vi "RunOperation.vi"(10 "Inputs":string[](array[string]), 11 "RunVIAnalyzer in":refnum<class "RunVIAnalyzer.lvclass">) -> (1 "Output/Failure":string, 2 "CLI Process Return Code":i32, 3 "RunVIAnalyzer out":refnum<class "RunVIAnalyzer.lvclass">)   [LabVIEW 2014, in "RunVIAnalyzer.lvclass"]
uses:
  RunVIAnalyzer.lvclass
  RunVIAnalyzer.lvclass/RunVIAnalyzer.ctl
  <vilib>/addons/analyzer/NI_VIAnalyzerTKVIs.lvlib
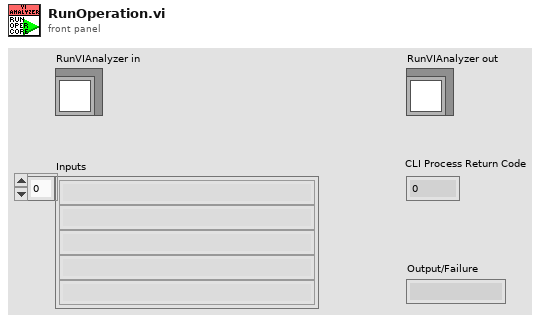
[diagram p1: front panel]
types:
  T1 = typedef "VIAnCtl Results.ctl" = cluster{"Test Name":string, "Results Data":T2[], "Status":T3, "Exceed Max Fails?":bool}
  T2 = typedef "VIAnCtl ResultsData (index).ctl" = cluster{"Result Message":string, "Ref Index":i32}
  T3 = typedef "VIAnCtl ResultStatus.ctl" = enum16{"Pass", "Fail", "Skipped", "VI not loadable", "Test not loadable", "Test not runnable", "Test error out"}
  T4 = typedef "VIAnRes Parsed Results Data (by VI).ctl" = cluster{"VI Path":path, "Pass":cluster{"row":i32, "column":i32}[], "Fail":cluster{"row":i32, "column":i32}[], "Skipped":cluster{"row":i32, "column":i32}[], "VI not loadable":cluster{"row":i32, "column":i32}[], "Test not loadable":cluster{"row":i32, "column":i32}[], "Test not runnable":cluster{"row":i32, "column":i32}[], "Test error out":cluster{"row":i32, "column":i32}[]}
  T5 = typedef "VIAnRes Parsed Results Data (by Test).ctl" = cluster{"Test Name":string, "Pass":cluster{"VI Path":path, "index":cluster{"row":i32, "column":i32}}[], "Fail":cluster{"VI Path":path, "index":cluster{"row":i32, "column":i32}}[], "Skipped":cluster{"VI Path":path, "index":cluster{"row":i32, "column":i32}}[]}
  T6 = typedef "VIAnCtl Test Config Data.ctl" = cluster{"Test Name":string, "Config Ref":refnum<vi>, "Ref Valid?":bool, "Test Ranking":T7, "Max Failures":u32, "Test Path":path, "Control Values":T8[], "Selected?":bool}
  T7 = typedef "VIAnCtl TestRanking.ctl" = u16
  T8 = typedef "VIAnCtl Config Control Value.ctl" = cluster{"Control Name":string, "Control Value":variant}
  T9 = cluster{"Raw Results":T1[][], "Parsed Results Data (by VI)":T4[], "Parsed Results Data (by Test)":T5[], "Summary Statistics":cluster{"Passed Tests":i32, "Failed Tests":i32, "Skipped Tests":i32, "VIs not loadable":i32, "Tests not loadable":i32, "Tests not runnable":i32, "Test error out":i32, "Start Time":u32, "Total Time (s)":dbl}, "Test Config Data":T6[]}
  T10 = cluster{"Passed Tests":i32, "Failed Tests":i32, "Skipped Tests":i32, "VIs not loadable":i32, "Tests not loadable":i32, "Tests not runnable":i32, "Test error out":i32, "Start Time":u32, "Total Time (s)":dbl}
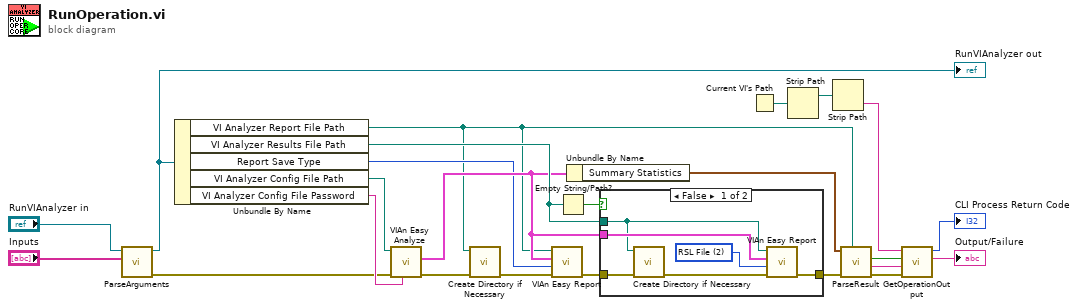
[diagram p0: block diagram]
diagram:
  n1 = call "ParseArguments.vi"("Inputs"="Inputs", "RunVIAnalyzer in"="RunVIAnalyzer in") -> ("error out"=w14:errorcluster, "RunVIAnalyzer out"=w24:refnum<class "RunVIAnalyzer.lvclass">)  [unwired: 8 in]
  "RunVIAnalyzer out" <- w24
  n2 = Unbundle By Name(w24) -> ("VI Analyzer Report File Path"=w1:path, "VI Analyzer Results File Path"=w5:path, "Report Save Type"=w3:u16, "VI Analyzer Config File Path"=w16:path, "VI Analyzer Config File Password"=w17:string)
  n3 = call <vilib>:"VIAn Easy Analyze.vi"("Configuration File Password"=w17, "error in (no error)"=w14, "Analysis Target"=w16) -> ("error out"=w18:errorcluster, "Analysis Results"=w4:T9)  [unwired: 7 in]
  n4 = call "Create Directory if Necessary.vi"("error in"=w18, "File Path"=w1) -> ("error out"=w2:errorcluster)  [unwired: 9 in]
  n5 = call <vilib>:"VIAn Easy Report.vi"("error in (no error)"=w2, "Report Save Type (ASCII)"=w3, "Analysis Results"=w4, "Report Save Path"=w1) -> ("error out"=w8:errorcluster)  [unwired: 7 in]
  n6 = Empty String/Path?(string/path=w5) -> (empty?=w6:bool)
  n7 = Unbundle By Name(w4) -> ("Summary Statistics"=w15:T10)
  n8 = case shown="False" w6 {
    tunnel: w8 -> [w27 w31]
    tunnel: [w30 w31] -> w7
    tunnel: w4 -> [w29 _]
    tunnel: w5 -> [w25 _]
    frame False {
      w28 = u16 2 items=["ASCII", "HTML", "RSL File"] ("Report Save Type (ASCII)")
      n9 = call "Create Directory if Necessary.vi"("error in"=w27, "File Path"=w25) -> ("error out"=w26:errorcluster)  [unwired: 9 in]
      n10 = call <vilib>:"VIAn Easy Report.vi"("error in (no error)"=w26, "Report Save Type (ASCII)"=w28, "Analysis Results"=w29, "Report Save Path"=w25) -> ("error out"=w30:errorcluster)  [unwired: 7 in]
    }
    frame True {
    }
  }
  n11 = Current VI's Path() -> (path=w21:path)
  n12 = Strip Path(path=w21) -> (stripped path=w20:path)  [unwired: 1 out]
  n13 = Strip Path(path=w20) -> (name=w19:string)  [unwired: 1 out]
  n14 = call "ParseResult.vi"("VI Analyzer report path"=w1, "error in (no error)"=w7, "Summary Statistics"=w15) -> ("error out"=w13:errorcluster, "Output"=w9:string, "Passed?"=w10:bool)  [unwired: 6 in]
  n15 = call "GetOperationOutput.vi"("error in (no error)"=w13, "Operation Output/Error In"=w9, "Operation succeeded?"=w10, "Operation Name"=w19) -> ("Operation Output/Error Out"=→"Output/Failure":string, "CLI Process Return Code"=→"CLI Process Return Code":i32)  [unwired: 6 in]
